vi "Durability_will_2012_07_05_pwm cahnges.vi"() -> ()   [LabVIEW 2011]
uses:
  <vilib>/DAQmx/write.llb/DAQmx Write (Counter Time 1Chan 1Samp).vi
  <vilib>/DAQmx/read.llb/DAQmx Read (Analog 1D Wfm NChan NSamp).vi
  <vilib>/measure/madcrms.llb/Basic Averaged DC-RMS for 1 Chan.vi
  <vilib>/DAQmx/miscellaneous.llb/DAQmx Fill In Error Info.vi
  <vilib>/Analysis/NI_AALBase.lvlib
  <vilib>/measure/NI_MAPro.lvlib
panel:
  out "Motor 1 Elapsed Time (s)":string caption="Elapsed Time Text"
  out "Motor 1 Start Time":string caption="Start Time Text"
  out "Motor 1 Down":bool
  out "Long Write":bool caption="Time has Elapsed"
  out "Short Write":bool caption="Time has Elapsed"
  out "Temps":dynamicdata(graph) caption="Signal Out"
  out "Power Graph":dynamicdata(graph) caption="Collected Signals"
  out "Errors":errorcluster
  out "RPM":dynamicdata(graph) caption="Collected Signals"
  out "Motor RPM":dbl format="%#.0f"
  out "Motor Power (watts)":dbl format="%#.4f"
  out "Power to MC1 (watts)":dbl format="%#.4f"
  out "Voltage to MC1 (volts)":dbl format="%#.4f"
  out "Current to MC1  (amps)":dbl format="%#.4f"
  in  "Manual Start":bool
  in  "Power \nSetting":i8(slide) min=0 max=100 step=10 scale=0.0..100.0
  out "Motor Temp (F)":dbl format="%.1f"
  out "Tank Temp (F)":dbl format="%.1f"
  in  "Quit 4":bool
  out "Phase to Phase Voltage":waveform(dbl)(graph)
  out "Phase Current":waveform(dbl)(graph)
  # "Temperature"
  # "MC1"
  # "Motor Power and RPM"
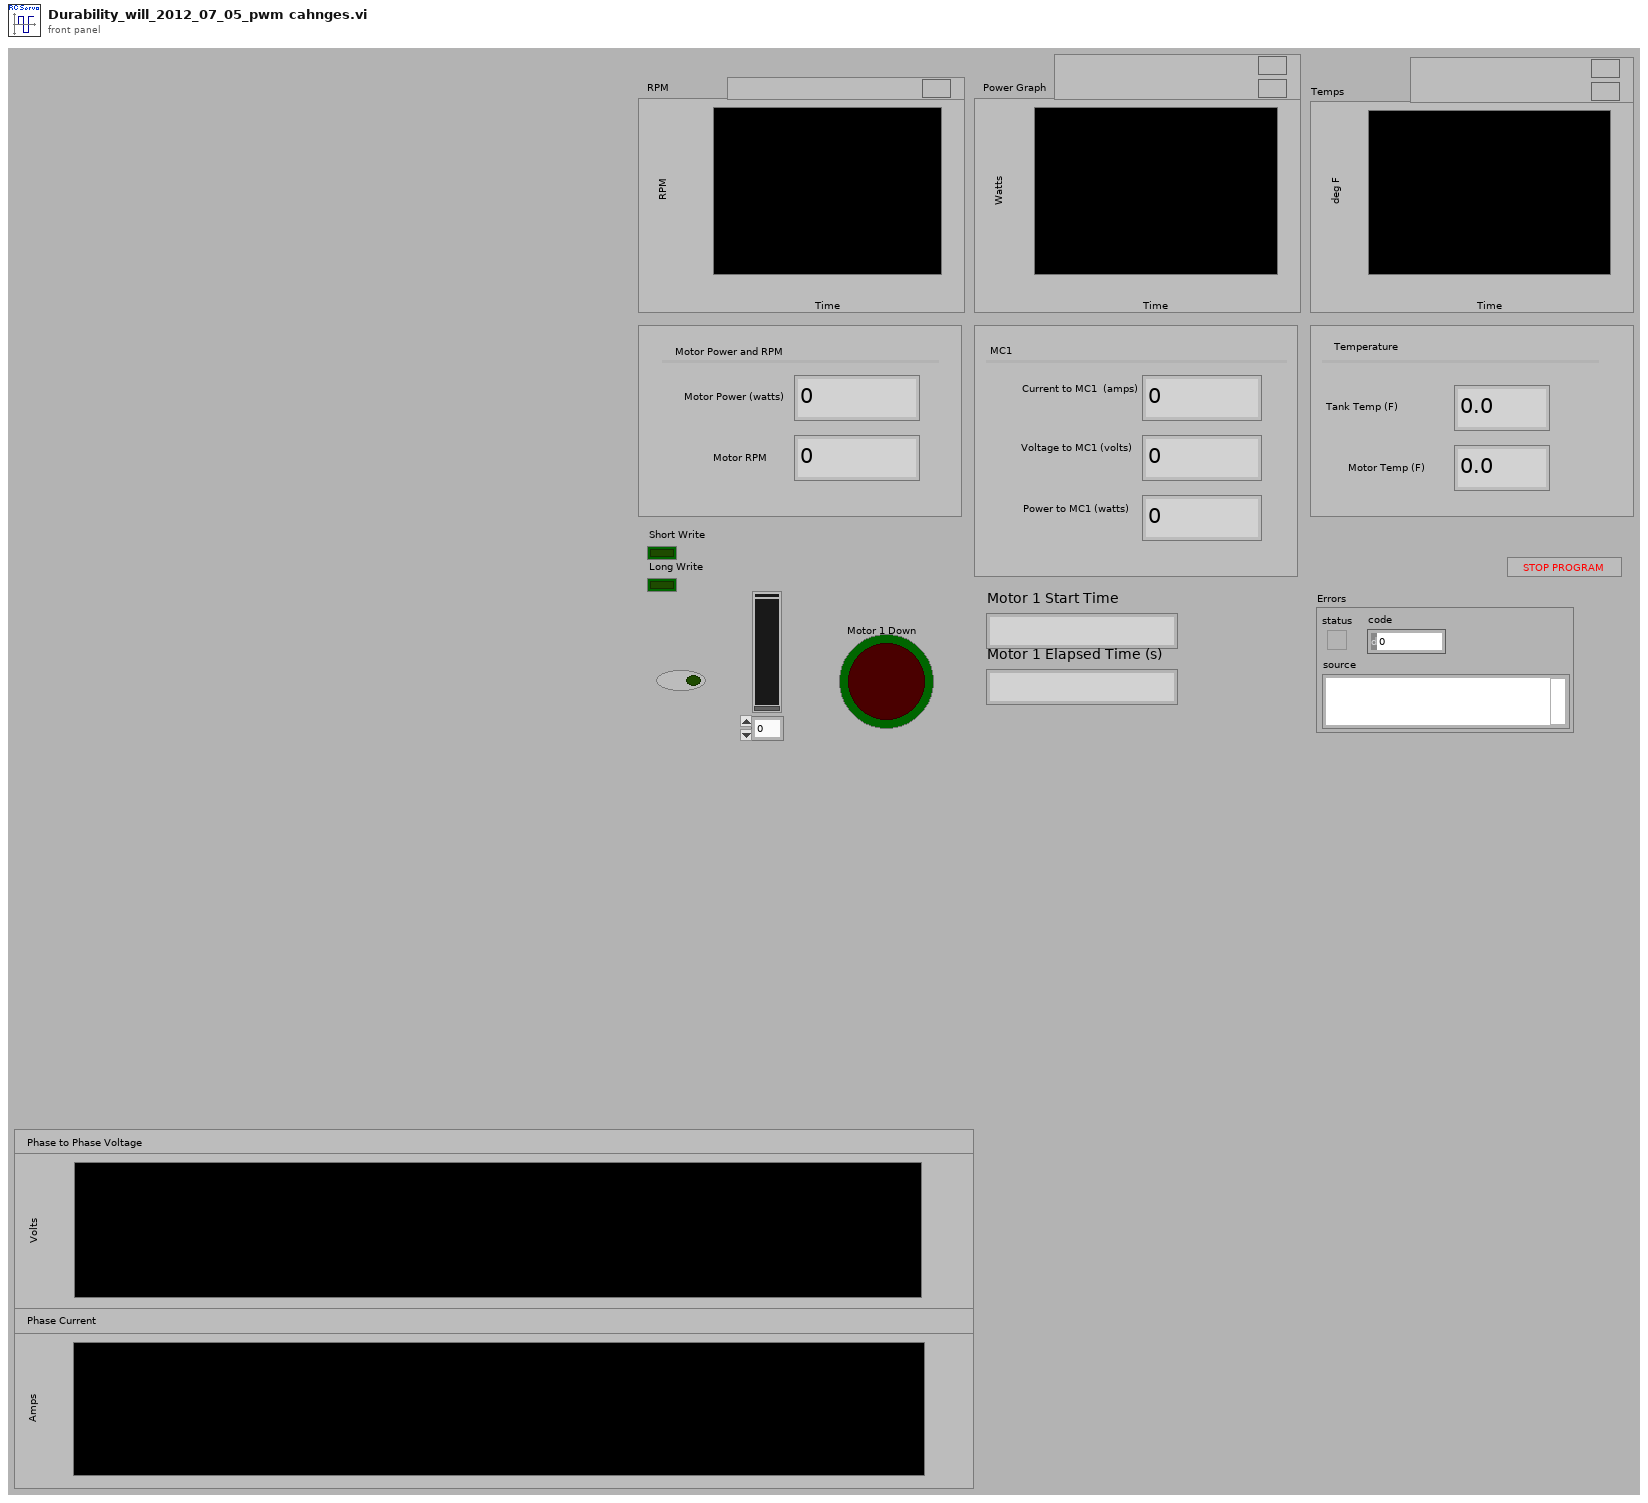
[diagram p1: front panel]
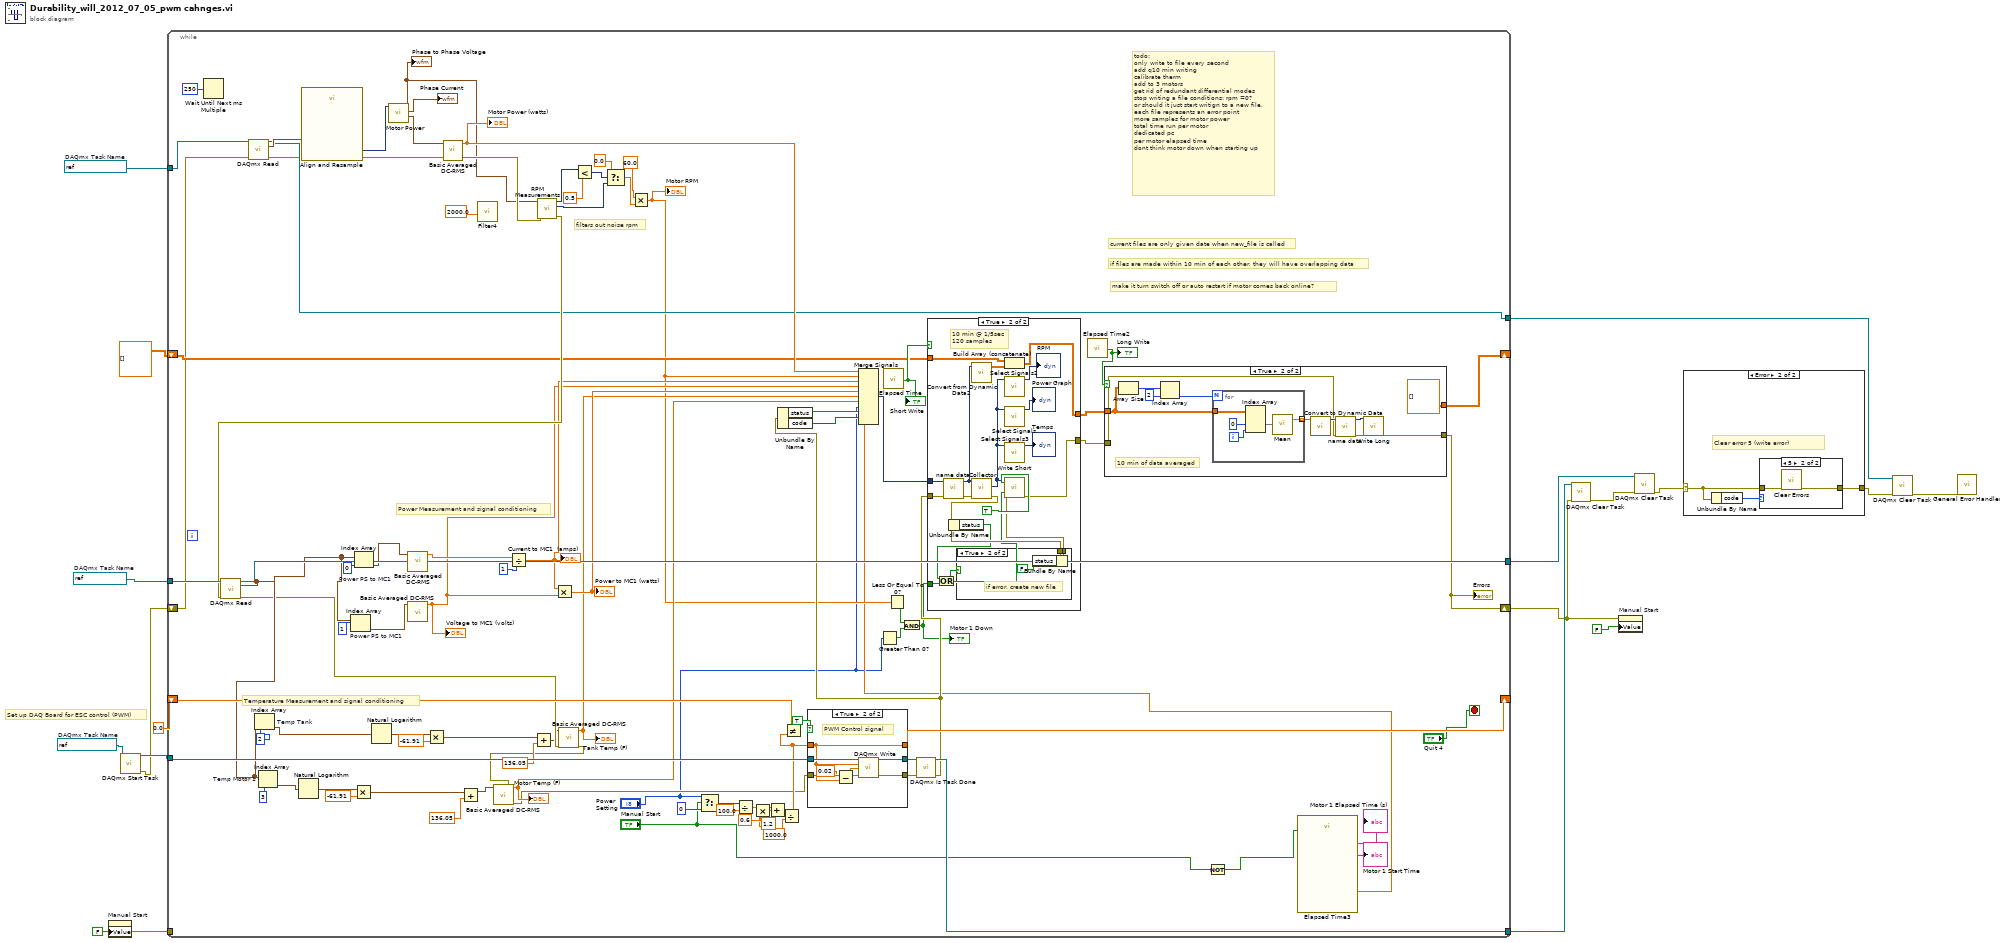
[diagram p0: block diagram]
diagram:
  w10 = refnum<k21> "PWM Signal"  # DAQmx Task Name
  w15 = refnum<k21> "MC Power"  # DAQmx Task Name
  w16 = refnum<k21> "Motor Power"  # DAQmx Task Name
  # "Set up DAQ Board for ESC control (PWM)"
  n1 = property on="Manual Start" class="Bool (strict)"("Value"=FALSE ("Run Motor")) -> (error out=w13:errorcluster)  [unwired: 2 in, 1 out]
  n2 = call <vilib>:"DAQmx Start Task.vi"("task/channels in"=w10) -> ("task out"=w9:refnum<k21>, "error out"=w1:errorcluster)  [unwired: 13 in]
  n3 = while {
    tunnel: [w108] -> w18
    tunnel: w9 -> [w107]
    shift-right: [w97] -> _
    shift-left: 0.0 -> [w100]
    tunnel: w15 -> [w92]
    tunnel: [w91] -> w17
    tunnel: [w40] -> w6
    tunnel: w16 -> [w81]
    tunnel: w13 -> [_]
    shift-right: [w43] -> _
    shift-left: dbl[][][] [] -> [w42]
    shift-right: [w39] -> w11
    shift-left: w1 -> [w36]
    stop <- "Quit 4" stop-if-true
    # "make it turn switch off or auto restart if motor comes back online?"
    # "if files are made within 10 min of each other, they will have overlapping data"
    # "current files are only given date when new_file is called"
    # "todo:\nonly write to file every second\nadd q10 min writing\ncalibrate therm\nadd to 3 motors\nget rid of redundant differential modes\nstop writing a file conditions: rpm =0?\nor should it just start writign to a new file,\neach file represents an error point\nmore samples for motor power\ntotal time run per motor\ndedicated pc\nper motor elapsed time\ndont think motor down when starting up"
    # "filters out noise rpm"
    # "Power Measurement and signal conditioning"
    # "Temperature Measurement and signal conditioning"
    n4 = Wait Until Next ms Multiple(millisecond multiple=u32 250) -> ()  [unwired: 1 out]
    n5 = call-poly <vilib>:"DAQmx Read.vi"("task/channels in"=w81, "error in"=w36) -> ("task out"=w40:refnum<k21>, "data"=w64:waveform(dbl)[], "error out"=w37:errorcluster)  [unwired: 11 in]
    n6 = call "Align and Resample"("Signals"=w64) -> ("Resampled Signals"=w65:dynamicdata)  [unwired: 8 in, 2 out]
    n7 = call "Motor Power.vi"("data"=w65) -> ("Waveform"=w58:waveform(dbl), "Phase Current"=→"Phase Current":waveform(dbl), "Phase to Phase Voltage"=w24:waveform(dbl))  [unwired: 7 in, 1 out]
    "Phase to Phase Voltage" <- w24
    n8 = call-poly <vilib>:"Basic Averaged DC-RMS.vi"("signal in"=w58) -> ("DC value"=w57:dbl)  [unwired: 7 in, 3 out]
    "Motor Power (watts)" <- w57
    n9 = call "Filter4"("Lower Cut-Off"=2000.0 ("LowPass Filter CutOff [Hz]")) -> ()  [unwired: 9 in, 2 out]
    n10 = call "RPM Measurements"("error in (no error)"=w37, "Signals"=w24) -> ("error out"=w80:errorcluster, "Frequency"=w86:dynamicdata, "Amplitude"=w83:dynamicdata)  [unwired: 7 in]
    n11 = call-poly <vilib>:"DAQmx Read.vi"("task/channels in"=w92, "error in"=w80) -> ("task out"=w91:refnum<k21>, "data"=w51:waveform(dbl)[], "error out"=w49:errorcluster)  [unwired: 11 in]
    n12 = Index Array "Temp Tank"(array=w51, index=2) -> (element=w52:waveform(dbl))
    n13 = Index Array "Temp Motor 1"(array=w51, index=3) -> (element=w75:waveform(dbl))
    n14 = Natural Logarithm(1:w75) -> (0:w79:waveform(dbl))
    n15 = Index Array "Power PS to MC1"(array=w51, index=1) -> (element=w54:waveform(dbl))
    n16 = Multiply(x=w79, y=-61.91) -> (x*y=w77:waveform(dbl))
    n17 = Index Array "Power PS to MC1"(array=w51, index=0) -> (element=w56:waveform(dbl))
    n18 = Natural Logarithm(1:w52) -> (0:w74:waveform(dbl))
    n19 = call-poly <vilib>:"Basic Averaged DC-RMS.vi"("signal in"=w56) -> ("DC value"=w55:dbl)  [unwired: 7 in, 3 out]
    n20 = call-poly <vilib>:"Basic Averaged DC-RMS.vi"("signal in"=w54) -> ("DC value"=w53:dbl)  [unwired: 7 in, 3 out]
    "Voltage to MC1 (volts)" <- w53
    n21 = Multiply(x=w74, y=-61.91) -> (x*y=w72:waveform(dbl))
    n22 = Add(x=w77, y=136.05) -> (x+y=w47:waveform(dbl))
    n23 = Divide(x=w55, y=1) -> (x/y=w69:dbl)
    "Current to MC1  (amps)" <- w69
    n24 = Add(x=w72, y=136.05) -> (x+y=w48:waveform(dbl))
    n25 = Multiply(x=w69, y=w53) -> (x*y=w68:dbl)
    "Power to MC1 (watts)" <- w68
    n26 = call-poly <vilib>:"Basic Averaged DC-RMS.vi"("error in (no error)"=w49, "signal in"=w48) -> ("error out"=w44:errorcluster, "DC value"=w50:dbl)  [unwired: 6 in, 2 out]
    "Tank Temp (F)" <- w50
    n27 = call-poly <vilib>:"Basic Averaged DC-RMS.vi"("error in (no error)"=w44, "signal in"=w47) -> ("error out"=w45:errorcluster, "DC value"=w46:dbl)  [unwired: 6 in, 2 out]
    "Motor Temp (F)" <- w46
    n28 = Less?(x=w83, y=0.5) -> (x < y?=w85:dynamicdata)
    n29 = Select(t=0.0, s=w85, f=w86) -> (s? t:f=w88:dbl)
    n30 = Multiply(x=60.0, y=w88) -> (x*y=w35:dbl)
    "Motor RPM" <- w35
    n31 = Select(t="Power \nSetting", s="Manual Start", f=i8 0) -> (s? t:f=w98:i8)
    n32 = Divide(x=w98, y=100.0) -> (x/y=w102:dbl)
    n33 = Multiply(x=w102, y=0.6 ("scale")) -> (x*y=w21:dbl)
    n34 = Add(x=w21, y=1.2 ("add")) -> (x+y=w22:dbl)
    n35 = Divide(x=w22, y=1000.0) -> (x/y=w101:dbl)
    n36 = Not Equal?(x=w100, y=w101) -> ()  [unwired: 1 out]
    n37 = case shown="True" TRUE {
      tunnel: w101 -> [w152 w156]
      tunnel: w107 -> [w153 w160]
      tunnel: [w153 w158] -> w106
      tunnel: [w151 w157] -> w105
      tunnel: [w152 w156] -> w97
      tunnel: w45 -> [w151 w155]
      frame False {
      }
      frame True {
        # "PWM Control signal"
        n38 = Subtract(x=0.02 ("total time"), y=w156) -> (x-y=w159:dbl)
        n39 = call-poly <vilib>:"DAQmx Write.vi"("task/channels in"=w160, "high time"=w156, "low time"=w159, "error in"=w155) -> ("task out"=w158:refnum<k21>, "error out"=w157:errorcluster)  [unwired: 9 in, 1 out]
      }
    }
    n40 = Greater Than 0?(x="Power \nSetting") -> (x > 0?=w33:bool)
    n41 = call "Elapsed Time"() -> ("Time has Elapsed"=w61:bool)  [unwired: 12 in, 7 out]
    "Short Write" <- w61
    n42 = Less Or Equal To 0?(x=w35) -> (x <= 0?=w34:bool)
    n43 = And(x=w34, y=w33) -> (x .and. y?=w32:bool)
    "Motor 1 Down" <- w32
    n44 = call <vilib>:"DAQmx Is Task Done.vi"("task/channels in"=w106, "error in"=w105) -> ("task out"=w108:refnum<k21>, "error out"=w62:errorcluster)  [unwired: 11 in, 1 out]
    n45 = Unbundle By Name(w62) -> ("status"=w67:bool, "code"=w66:i32)
    n46 = call "Elapsed Time2"() -> ("Time has Elapsed"=w60:bool)  [unwired: 12 in, 7 out]
    "Long Write" <- w60
    n47 = Not(x="Manual Start") -> (.not. x?=w28:bool)
    n48 = call "Elapsed Time3"("Reset"=w28) -> ("Start Time Text"=→"Motor 1 Start Time":string, "Elapsed Time (s)"=w27:dbl, "Elapsed Time Text"=→"Motor 1 Elapsed Time (s)":string)  [unwired: 11 in, 5 out]
    n49 = Merge Signals(w57, w35, w69, w53, w68, w50, w46, "Power \nSetting", w67, w66, w27) -> (w59:dynamicdata)
    n50 = case shown="True" w61 {
      tunnel: w59 -> [_ w142]
      tunnel: w62 -> [w128 w139]
      tunnel: [w128 w134] -> w38
      tunnel: [w127 w146] -> w41
      tunnel: w42 -> [w127 w145]
      tunnel: w32 -> [_ w130]
      frame False {
      }
      frame True {
        # "10 min @ 1/5sec\n120 samples"
        n51 = call "name data.vi"("error in (no error)"=w139, "Dynamic Data"=w142) -> ("error out"=w140:errorcluster, "Output"=w141:dynamicdata)  [unwired: 8 in]
        n52 = call "Convert from Dynamic Data2"("Dynamic Data Type"=w141) -> ("Array"=w144:dbl[][])  [unwired: 3 in]
        n53 = call "Collector"("error in (no error)"=w140, "Signals"=w141) -> ("error out"=w132:errorcluster, "Collected Signals"=w135:dynamicdata)  [unwired: 8 in]
        n54 = Unbundle By Name(w132) -> ("status"=w131:bool)
        n55 = Or(x=w131, y=w130) -> (x .or. y?=w129:bool)
        n56 = case shown="True" w129 {
          tunnel: [w147 w150] -> w133
          tunnel: w132 -> [w147 w149]
          frame False {
          }
          frame True {
            # "if error, create new file"
            n57 = Bundle By Name(cluster=w149, "status"=FALSE) -> (w150:errorcluster)
          }
        }
        n58 = Build Array (concatenate)(w145, w144) -> (w146:dbl[][][])
        n59 = call "Select Signals2"("Signals"=w135) -> ("Signal Out"=→"RPM":dynamicdata)  [unwired: 9 in, 1 out]
        n60 = call "Select Signals"("Signals"=w135) -> ("Signal Out"=→"Power Graph":dynamicdata)  [unwired: 9 in, 1 out]
        n61 = call "Select Signals3"("Signals"=w135) -> ("Signal Out"=→"Temps":dynamicdata)  [unwired: 9 in, 1 out]
        n62 = call "Write Short"("Signals"=w135, "Reset"=TRUE, "new_file"=w129, "error in (no error)"=w133) -> ("error out"=w134:errorcluster)  [unwired: 13 in, 2 out]
      }
    }
    n63 = case shown="True" w60 {
      tunnel: w41 -> [w110 w121]
      tunnel: [w110 dbl[][][] []] -> w43
      tunnel: w38 -> [w109 w113]
      tunnel: [w109 w111] -> w39
      frame False {
      }
      frame True {
        # "10 min of data averaged"
        n64 = Array Size(array=w121) -> (size(s)=w117:i32[])
        n65 = Index Array(array=w117, index=2) -> (element=w118:i32)
        n66 = for {
          N: w118 -> [_]
          tunnel: w121 -> [w126]
          tunnel: [w122] -> w116 mode=indexing
          i -> [w125]
          n67 = Index Array(array=w126, index (dim 1)=0 ("disabled index (row)"), index (dim 2)=w125) -> (element=w124:dbl[])  [unwired: 1 in]
          n68 = call <vilib>:"Mean.vi"("X"=w124) -> ("mean"=w122:dbl)  [unwired: 1 out]
        }
        n69 = call "Convert to Dynamic Data"("Array"=w116) -> ("Dynamic Data Type"=w115:dynamicdata)  [unwired: 3 in]
        n70 = call "name data.vi"("error in (no error)"=w113, "Dynamic Data"=w115) -> ("error out"=w112:errorcluster, "Output"=w114:dynamicdata)  [unwired: 8 in]
        n71 = call "Write Long"("Signals"=w114, "error in (no error)"=w112) -> ("error out"=w111:errorcluster)  [unwired: 15 in, 2 out]
      }
    }
    "Errors" <- w39
  }
  n72 = call <vilib>:"DAQmx Clear Task.vi"("task in"=w18, "error in"=w11) -> ("error out"=w2:errorcluster)  [unwired: 13 in]
  n73 = property on="Manual Start" class="Bool (strict)"(error in=w11, "Value"=FALSE ("Run Motor")) -> ()  [unwired: 1 in, 2 out]
  n74 = call <vilib>:"DAQmx Clear Task.vi"("task in"=w17, "error in"=w2) -> ("error out"=w4:errorcluster)  [unwired: 13 in]
  n75 = case shown="Error" w4 {
    selector: w4 -> [w161 w163]
    tunnel: [w161 w162] -> w3
    frame No Error {
    }
    frame Error {
      # "Clear error 5 (write error)"
      n76 = Unbundle By Name(w163) -> ("code"=w164:i32)
      n77 = case shown="5" w164 {
        tunnel: w163 -> [w165 w167]
        tunnel: [w165 w166] -> w162
        frame Default {
        }
        frame 5 {
          n78 = call <vilib>:"Clear Errors.vi"("error in (no error)"=w167) -> ("error out"=w166:errorcluster)  [unwired: 6 in]
        }
      }
    }
  }
  n79 = call <vilib>:"DAQmx Clear Task.vi"("task in"=w6, "error in"=w3) -> ("error out"=w5:errorcluster)  [unwired: 13 in]
  n80 = call <vilib>:"General Error Handler.vi"("error in (no error)"=w5) -> ()  [unwired: 10 in, 5 out]
